vi "Interpret_JSON.vi"(6 "Server VI":refnum<vi>, 7 "Direction":enum16{"ASK", "TELL"}(ring), 8 "error in (no error)":errorcluster, 10 "payload":string, 11 "Command":string) -> (0 "error out":errorcluster, 1 "Send to Server":string, 3 "Read from Server":string)   [LabVIEW 2020]
uses:
  JSON_Formats.vi
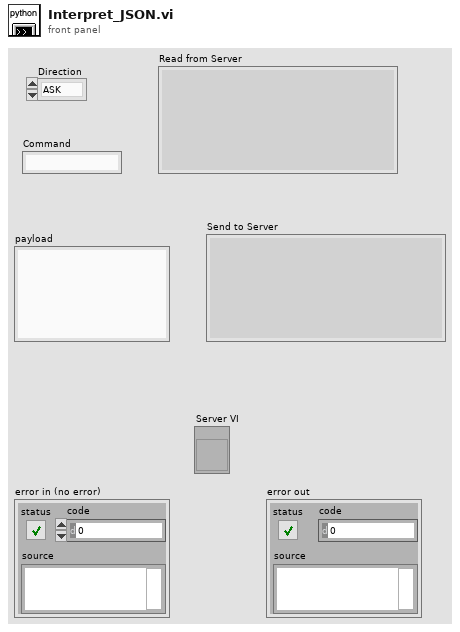
[diagram p1: front panel]
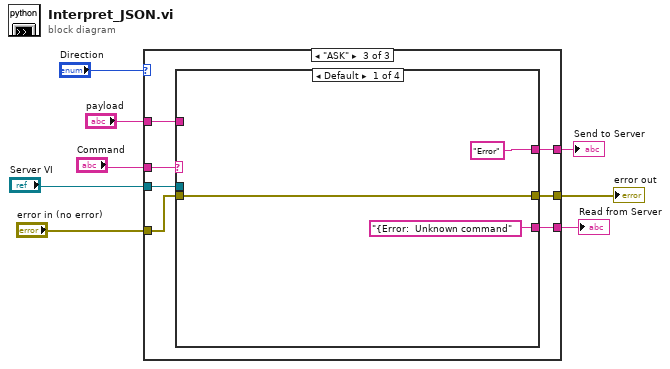
[diagram p0: block diagram]
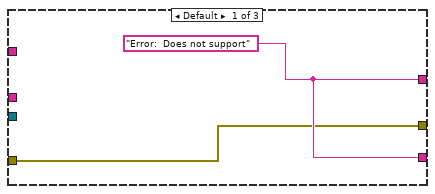
[diagram p2: hidden frame]
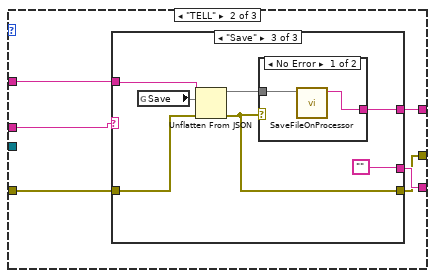
[diagram p3: hidden frame]
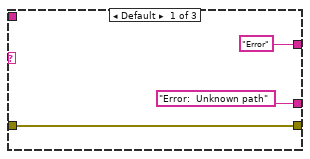
[diagram p4: hidden frame]
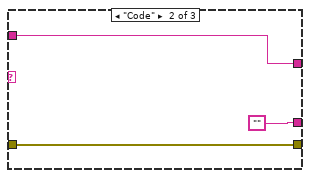
[diagram p5: hidden frame]
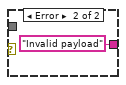
[diagram p6: hidden frame]
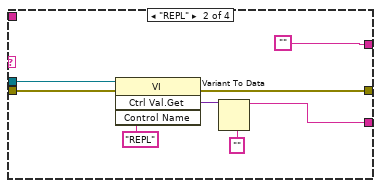
[diagram p7: hidden frame]
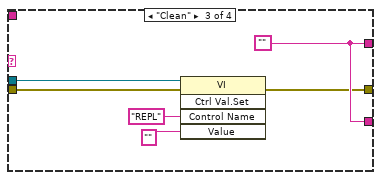
[diagram p8: hidden frame]
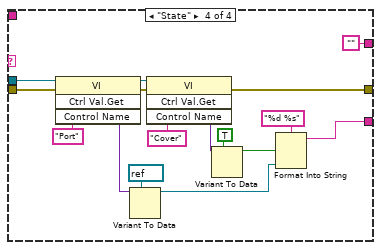
[diagram p9: hidden frame]
diagram:
  n1 = case shown="\"ASK\"" "Direction" {
    tunnel: [w10 w16 w39] -> w8
    tunnel: "payload" -> [_ w15 w38]
    tunnel: [w10 w14 w37] -> w6
    tunnel: "Server VI" -> [_ _ w36]
    tunnel: "error in (no error)" -> [w9 w13 w35]
    tunnel: [w9 w12 w34] -> w5
    tunnel: "Command" -> [_ w11 w33]
    frame Default {
      w10 = "Error:  Does not support" ("input 2")
    }
    frame "TELL" {
      n2 = case shown="\"Save\"" w11 {
        tunnel: ["Error:  Unknown path" ("input 2") "" ""] -> w16
        tunnel: w15 -> [_ w21 w29]
        tunnel: ["Error" ("input 2") w21 w27] -> w14
        tunnel: w13 -> [w17 w20 w25]
        tunnel: [w17 w20 w24] -> w12
        frame Default {
        }
        frame "Code" {
        }
        frame "Save" {
          n3 = global read "JSON_Formats.vi" "Save"() -> (w26)
          n4 = Unflatten From JSON(JSON string=w29, type and defaults=w26, error in (no error)=w25) -> (value=w28, error out=w24:errorcluster)  [unwired: 4 in]
          n5 = case shown="No Error" w24 {
            tunnel: w28 -> [w31 _]
            tunnel: [w30 "Invalid payload" ("Code")] -> w27
            frame No Error {
              n6 = call "SaveFileOnProcessor.vi"("Save"=w31) -> ("Code"=w30:string)  [unwired: 10 in]
            }
            frame Error {
            }
          }
        }
      }
    }
    frame "ASK" {
      n7 = case shown="Default" w33 {
        tunnel: ["{Error:  Unknown command" ("input 2") w43 w56 w57] -> w39
        tunnel: w38 -> [_ _ _ _]
        tunnel: ["Error" ("input 2") "" w56 ""] -> w37
        tunnel: w36 -> [_ w45 w53 w68]
        tunnel: w35 -> [w40 w46 w52 w67]
        tunnel: [w40 w44 w51 w65] -> w34
        frame Default {
        }
        frame "REPL" {
          n8 = invoke class="VI" method="Ctrl Val.Get"(reference=w45, error in=w46, "Control Name"="REPL") -> (error out=w44:errorcluster, "Get Control Value Variant"=w48:variant)  [unwired: 1 in, 2 out]
          n9 = Variant To Data(type="" ("Control Name"), Variant=w48) -> (data=w43:string)  [unwired: 1 in, 1 out]
        }
        frame "Clean" {
          w56 = ""
          n10 = invoke class="VI" method="Ctrl Val.Set"(reference=w53, error in=w52, "Control Name"="REPL", "Value"="" ("Control Name")) -> (error out=w51:errorcluster)  [unwired: 1 in, 4 out]
        }
        frame "State" {
          n11 = invoke class="VI" method="Ctrl Val.Get"(reference=w68, error in=w67, "Control Name"="Port") -> (reference out=w66:refnum<vi>, error out=w69:errorcluster, "Get Control Value Variant"=w62:variant)  [unwired: 1 in, 1 out]
          n12 = Variant To Data(type=refnum<visa-resource-name> refnum ("Port"), Variant=w62) -> (data=w58:refnum<visa-resource-name>)  [unwired: 1 in, 1 out]
          n13 = invoke class="VI" method="Ctrl Val.Get"(reference=w66, error in=w69, "Control Name"="Cover") -> (error out=w65:errorcluster, "Get Control Value Variant"=w61:variant)  [unwired: 1 in, 2 out]
          n14 = Variant To Data(type=TRUE, Variant=w61) -> (data=w60:bool)  [unwired: 1 in, 1 out]
          n15 = Format Into String(format string="%d %s", w60, w58) -> (resulting string=w57:string)  [unwired: 2 in, 1 out]
        }
      }
    }
  }
  "Read from Server" <- w8
  "Send to Server" <- w6
  "error out" <- w5
